vi "Write Arm.vi"(8 "error in (no error)":errorcluster, 10 "Arm":refnum<data-value>, 11 "Fault-Injection Bus in":refnum<class "Fault-Injection Bus.lvclass">) -> (0 "error out":errorcluster, 3 "Fault-Injection Bus out":refnum<class "Fault-Injection Bus.lvclass">)   [LabVIEW 2021, in "Fault-Injection Bus.lvclass"]
uses:
  Fault-Injection Bus.lvclass
  Fault-Injection Bus.lvclass/Fault-Injection Bus.ctl
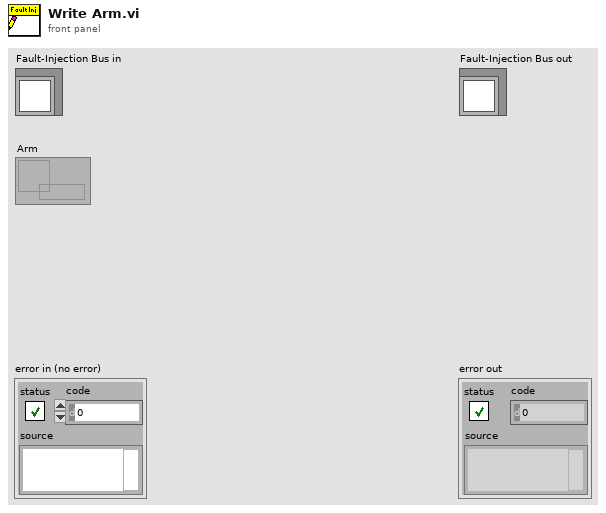
[diagram p1: front panel]
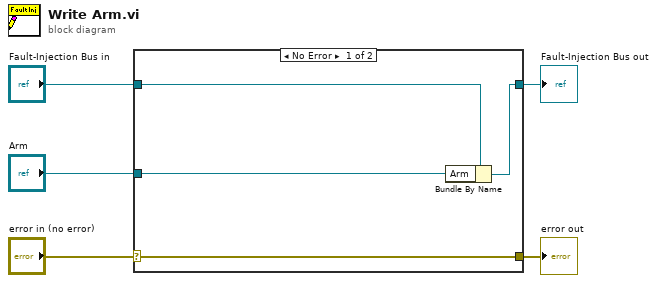
[diagram p0: block diagram]
diagram:
  n1 = case shown="No Error" "error in (no error)" {
    selector: "error in (no error)" -> [w9 w10]
    tunnel: [w9 w10] -> w4
    tunnel: [w7 w11] -> w2
    tunnel: "Fault-Injection Bus in" -> [w8 w11]
    tunnel: "Arm" -> [w6 _]
    frame No Error {
      n2 = Bundle By Name(cluster=w8, "Arm"=w6) -> (w7:refnum<class "Fault-Injection Bus.lvclass">)
    }
    frame Error {
    }
  }
  "error out" <- w4
  "Fault-Injection Bus out" <- w2
